vi "Save to file.vi"(8 "error in (no error)":errorcluster, 11 "Loop Data":T1) -> (0 "error out":errorcluster)   [LabVIEW 2015]
uses:
  TypDefs/Loop Data.ctl
  <vilib>/Utility/file.llb/Write Delimited Spreadsheet (DBL).vi
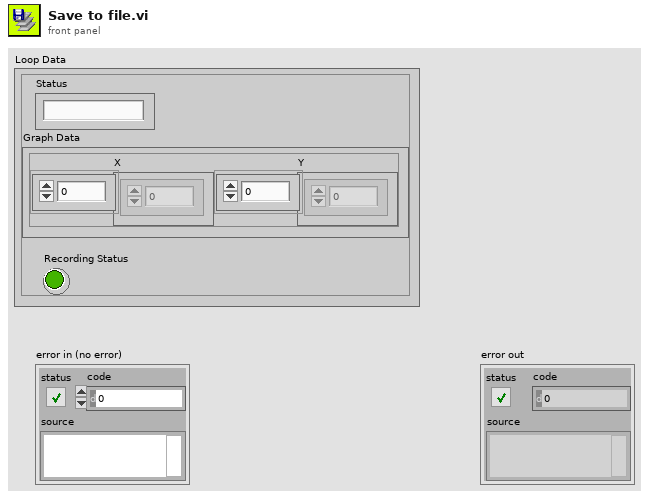
[diagram p1: front panel]
types:
  T1 = typedef "Loop Data.ctl" = cluster{"Status":string, "Graph Data":cluster{"X":dbl[], "Y":dbl[]}, "Recording Status":bool}
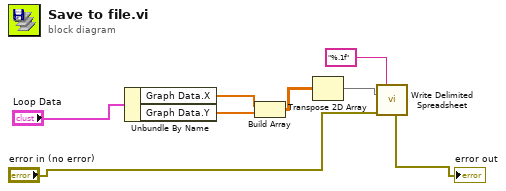
[diagram p0: block diagram]
diagram:
  n1 = Unbundle By Name("Loop Data") -> ("Graph Data.X"=w6:dbl[], "Graph Data.Y"=w5:dbl[])
  n2 = Build Array(w6, w5) -> (w1:dbl[][])
  n3 = Transpose 2D Array(2D array=w1) -> (transposed array=w2:dbl[][])
  n4 = call-poly <vilib>:"Write Delimited Spreadsheet.vi"("format (%.3f)"="%.1f", "2D data"=w2, "error in (no error)"="error in (no error)") -> ("error out"=→"error out":errorcluster)  [unwired: 11 in, 1 out]
